vi "Obtain Module Semaphore.vi"(8 "error in":errorcluster) -> (0 "error out":errorcluster, 1 "created new":bool, 3 "semaphore":T1)   [LabVIEW 2024, in "Chart.lvlib"]
doc: "Obtain the module semaphore reference.\n_____\nCreated using DQMH Event Scripter 6.1.0.128."
uses:
  Chart.lvlib
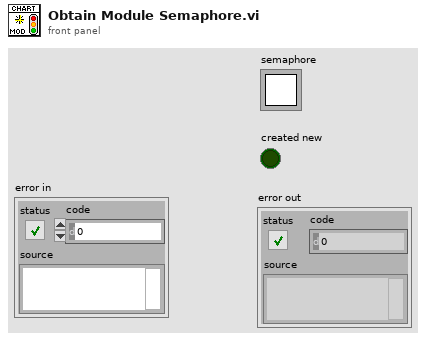
[diagram p1: front panel]
types:
  T1 = typedef "Semaphore RefNum" = refnum<k1>
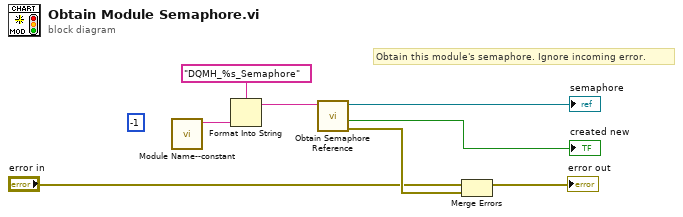
[diagram p0: block diagram]
diagram:
  (unwired) -1 ("Module ID")
  # "Obtain this module's semaphore. Ignore incoming error."
  n1 = call "Module Name--constant.vi"() -> ("Module Name"=w2:string)  [unwired: 11 in]
  n2 = Format Into String(format string="DQMH_%s_Semaphore", w2) -> (resulting string=w7:string)  [unwired: 2 in, 1 out]
  n3 = call <vilib>:"Obtain Semaphore Reference.vi"("name (unnamed)"=w7) -> ("error out"=w5:errorcluster, "created new"=→"created new":bool, "semaphore"=→"semaphore":T1)  [unwired: 4 in]
  n4 = Merge Errors("error in", w5) -> (→"error out":errorcluster)
